vi "load_list_of_presets.vi"(8 "error in (no error)":errorcluster, 11 "ColorOverlay in":refnum<class "ColorOverlay.lvclass">) -> (0 "error out":errorcluster, 3 "ColorOverlay out":refnum<class "ColorOverlay.lvclass">)   [LabVIEW 2010, in "ColorOverlay.lvclass"]
uses:
  ColorOverlay.lvclass
  ColorOverlay.lvclass/ColorOverlay.ctl
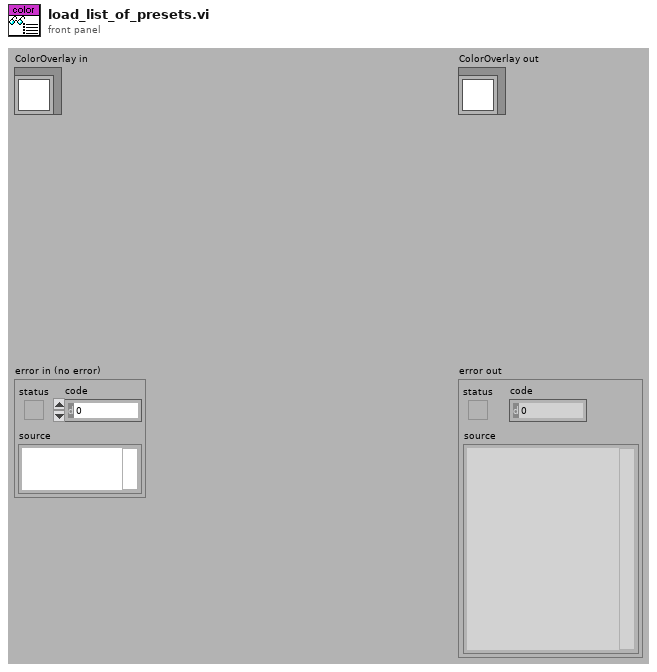
[diagram p1: front panel]
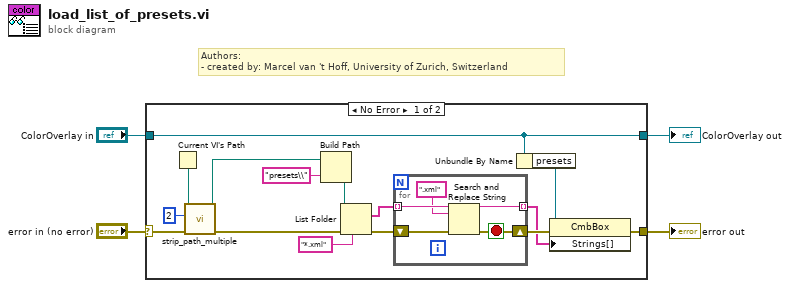
[diagram p0: block diagram]
diagram:
  # "Authors: \n- created by: Marcel van 't Hoff, University of Zurich, Switzerland"
  n1 = case shown="No Error" "error in (no error)" {
    selector: "error in (no error)" -> [w19 w26]
    tunnel: [w17 w26] -> w3
    tunnel: [w18 w25] -> w1
    tunnel: "ColorOverlay in" -> [w18 w25]
    frame No Error {
      n2 = Current VI's Path() -> (path=w16:path)
      n3 = call "strip_path_multiple.vi"("error in (no error)"=w19, "number of strips"=2, "path in"=w16) -> ("error out"=w11:errorcluster, "path out"=w14:path)  [unwired: 7 in]
      n4 = Build Path(base path=w14, name or relative path="presets\\") -> (appended path=w12:path)
      n5 = List Folder(path=w12, pattern="*.xml", error in=w11) -> (filenames=w10:string[], error out=w9:errorcluster)  [unwired: 1 in, 2 out]
      n6 = for {
        tunnel: w10 -> [w24] mode=indexing
        shift-right: [w22] -> w7
        shift-left: w9 -> [w23]
        tunnel: [w21] -> w5 mode=indexing
        stop <- w22 stop-if-true
        n7 = Search and Replace String(input string=w24, search string=".xml" ("pattern"), error in=w23) -> (result string=w21:string, error out=w22:errorcluster)  [unwired: 5 in, 2 out]
      }
      n8 = Unbundle By Name(w18) -> ("presets"=w6:refnum<vi>)
      n9 = property class="CmbBox"(reference=w6, error in=w7, "Strings[]"=w5) -> (error out=w17:errorcluster)  [unwired: 1 out]
    }
    frame Error {
    }
  }
  "error out" <- w3
  "ColorOverlay out" <- w1
